vi "LoadControlPanel.vi"(8 "error in (no error)":errorcluster, 10 "Actor In":refnum<class "Actor.lvclass">, 11 "GRMActor in":refnum<class "GeneralRMActor.lvclass">) -> (0 "error out":errorcluster, 3 "GRMActor out":refnum<class "GeneralRMActor.lvclass">)   [LabVIEW 2020, in "GeneralRMActor.lvlib" / "GeneralRMActor.lvclass"]
uses:
  GeneralRMActor.lvclass
  C:/Program Files/National Instruments/LabVIEW 2020/vi.lib/ActorFramework/Actor/Actor.lvclass
  <vilib>/ActorFramework/Actor/Actor.lvclass
  GeneralRMActor.lvclass/GeneralRMActor.ctl
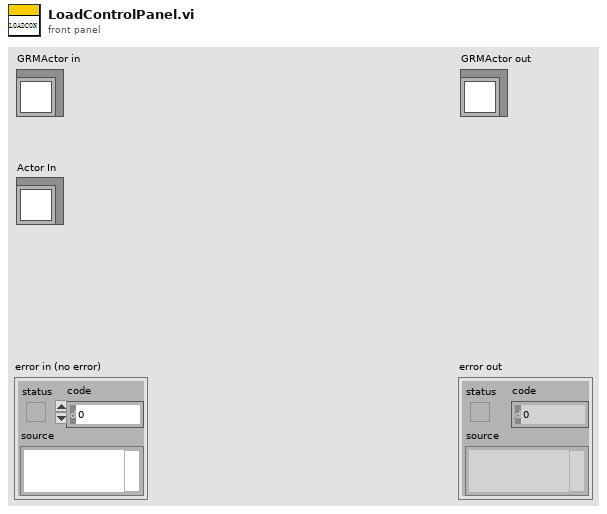
[diagram p1: front panel]
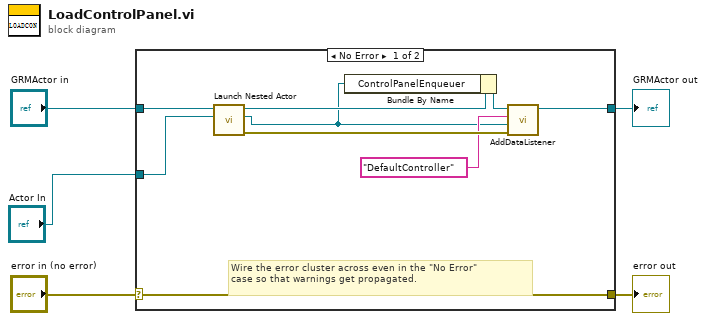
[diagram p0: block diagram]
diagram:
  n1 = case shown="No Error" "error in (no error)" {
    selector: "error in (no error)" -> [w14 w16]
    tunnel: [w14 w16] -> w4
    tunnel: [w9 w15] -> w2
    tunnel: "GRMActor in" -> [w10 w15]
    tunnel: "Actor In" -> [w11 _]
    frame No Error {
      # "Wire the error cluster across even in the \"No Error\"\ncase so that warnings get propagated."
      n2 = call <vilib>:"Launch Nested Actor.vi"("Nested Actor"=w11, "Caller Actor in"=w10) -> ("error out"=w13:errorcluster, "Nested Actor's Enqueuer"=w6:refnum<class "Message Enqueuer.lvclass">, "Caller Actor out"=w8:refnum<class "GeneralRMActor.lvclass">)  [unwired: 7 in]
      n3 = Bundle By Name(cluster=w8, "ControlPanelEnqueuer"=w6) -> (w7:refnum<class "GeneralRMActor.lvclass">)
      n4 = call-dynamic "AddDataListener.vi"("error in (no error)"=w13, "Listener In"=w6, "Label"="DefaultController", "GRMActor in"=w7) -> ("GRMActor out"=w9:refnum<class "GeneralRMActor.lvclass">)  [unwired: 6 in, 1 out]
    }
    frame Error {
    }
  }
  "error out" <- w4
  "GRMActor out" <- w2
